vi "myRIO_BRig_RT_TCP__buildStr_initTrial.vi"(7 "input_countTrial":u16, 9 "input_spout":enum16{"Left", "Right"}(ring), 10 "input_iTrial":u16, 11 "input_iBlock":u16) -> (3 "output_str_initTrial":string)   [LabVIEW 2014]
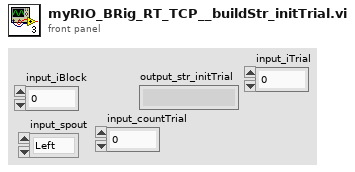
[diagram p1: front panel]
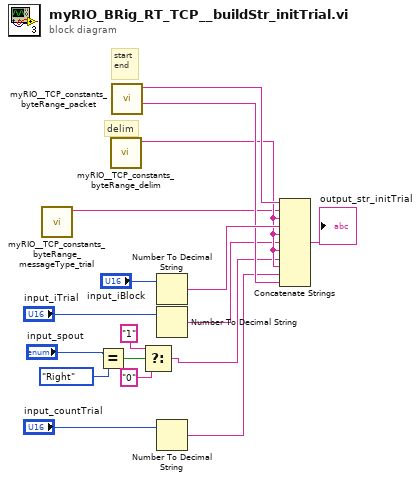
[diagram p0: block diagram]
diagram:
  # "start\nend"
  # "delim"
  n1 = call "myRIO__TCP_constants_byteRange_messageType_trial.vi"() -> ("output_Trial_char"=w7:string)  [unwired: 10 in, 1 out]
  n2 = Equal?(x="input_spout", y=enum16{"Left", "Right"}."Right") -> (x = y?=w5:bool)
  n3 = call "myRIO__TCP_constants_byteRange_delim.vi"() -> ("output_delim_char"=w11:string)  [unwired: 10 in, 1 out]
  n4 = call "myRIO__TCP_constants_byteRange_packet.vi"() -> ("output_end_char"=w13:string, "output_start_char"=w15:string)  [unwired: 8 in, 2 out]
  n5 = Select(t="1", s=w5, f="0") -> (s? t:f=w1:string)
  n6 = Number To Decimal String(number="input_iBlock") -> (decimal integer string=w17:string)  [unwired: 1 in]
  n7 = Number To Decimal String(number="input_iTrial") -> (decimal integer string=w8:string)  [unwired: 1 in]
  n8 = Number To Decimal String(number="input_countTrial") -> (decimal integer string=w12:string)  [unwired: 1 in]
  n9 = Concatenate Strings(w15, w7, w11, w17, w11, w8, w11, w1, w11, w12, w13) -> (→"output_str_initTrial":string)
